vi "destroy context.vi"(8 "error in (no error)":errorcluster, 11 "Communication Channel in":refnum<class "Communication Channel.lvclass">) -> (0 "error out":errorcluster, 3 "Communication Channel out":refnum<class "Communication Channel.lvclass">)   [LabVIEW 2018, in "Communication Channel.lvclass"]
uses:
  Communication Channel.lvclass
  Communication Channel.lvclass/Communication Channel.ctl
  Socket2/Socket2/Socket2.lvclass
  <vilib>/addons/zeromq/zmq_context.lvclass
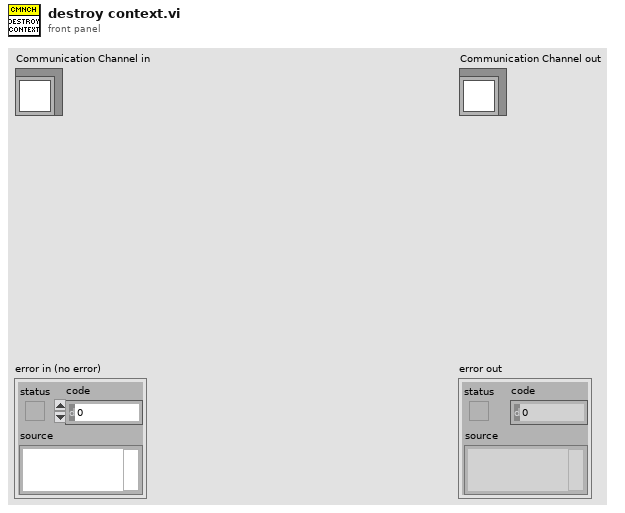
[diagram p1: front panel]
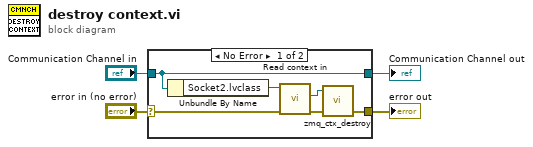
[diagram p0: block diagram]
diagram:
  n1 = case shown="No Error" "error in (no error)" {
    selector: "error in (no error)" -> [w8 w12]
    tunnel: [w5 w12] -> w3
    tunnel: [w10 w11] -> w1
    tunnel: "Communication Channel in" -> [w10 w11]
    frame No Error {
      n2 = Unbundle By Name(w10) -> ("Socket2.lvclass"=w9:refnum<class "Socket2.lvclass">)
      n3 = call-dynamic "Read context in.vi"("error in (no error)"=w8, "Socket2 in"=w9) -> ("error out"=w7:errorcluster, "zeromq.lvlib:ZeroMQ Context"=w6:refnum<class "zmq_context.lvclass">)  [unwired: 7 in, 1 out]
      n4 = call <vilib>:"zmq_ctx_destroy.vi"("error in"=w7, "context in"=w6) -> ("error out"=w5:errorcluster)  [unwired: 3 in]
    }
    frame Error {
    }
  }
  "error out" <- w3
  "Communication Channel out" <- w1
